vi "Proyecto_KevinLopez.vi"() -> ()   [LabVIEW 2020]
uses:
  <vilib>/userDefined/High Color/IMAQdx.ctl
  <vilib>/vision/driver/NI_Vision_Acquisition_Software.lvlib
  <vilib>/vision/NI_Vision_Development_Module.lvlib
panel:
  out "Amarillo":bool
  out "Rojo":bool
  out "Azul":bool
  out "Verde":bool
  out "Color Spectrum":dbl[](array[numeric]) format="%.2f"
  in  "Color Sensitivity":u32(ring) items=["Low", "Medium", "High"]
  in  "Session In":T1
  in  "stop":bool
  out "Image":T2(plugin-control)
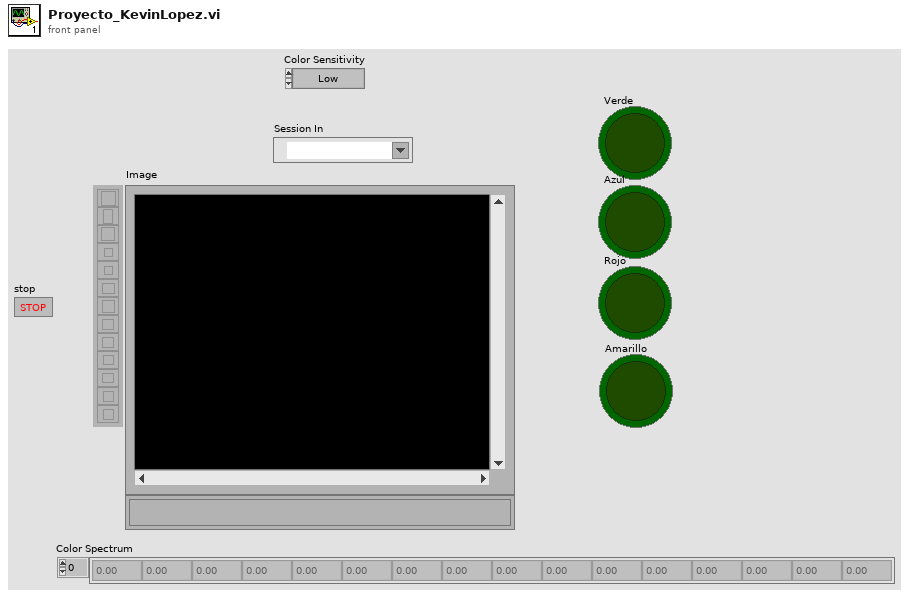
[diagram p1: front panel]
types:
  T1 = typedef "IMAQdx.ctl" = refnum<k21>
  T2 = typedef "IMAQ Image.ctl" = refnum<image>
  T3 = cluster{"Global Rectangle":i32[], "Contours":cluster{"Contour Type":u32, "ROI Type":u32, "Points":i32[]}[]}
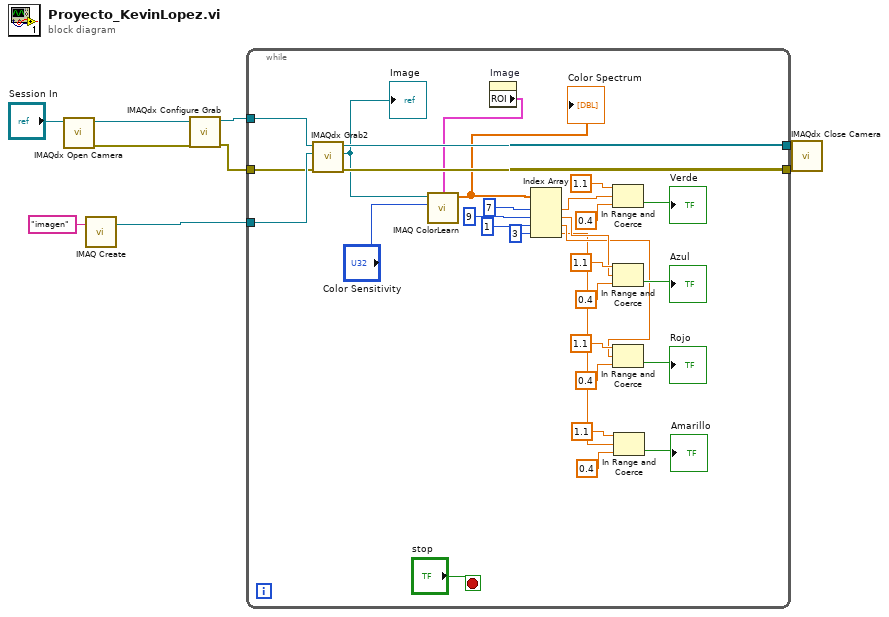
[diagram p0: block diagram]
diagram:
  n1 = call <vilib>:"IMAQdx Open Camera.vi"("Session In"="Session In") -> ("error out"=w8:errorcluster, "Session Out"=w9:T1)  [unwired: 9 in]
  n2 = call "IMAQ Create"("Image Name"="imagen") -> ("New Image"=w6:T2)  [unwired: 4 in, 1 out]
  n3 = call <vilib>:"IMAQdx Configure Grab.vi"("error in"=w8, "Session In"=w9) -> ("error out"=w5:errorcluster, "Session Out"=w4:T1)  [unwired: 8 in]
  n4 = while {
    tunnel: w6 -> [w39]
    tunnel: w5 -> [w38]
    tunnel: w4 -> [w37]
    tunnel: [w34] -> w3
    tunnel: [w36] -> w2
    stop <- "stop" stop-if-true
    n5 = call <vilib>:"IMAQdx Grab2.vi"("error in"=w38, "Image In"=w39, "Session In"=w37) -> ("error out"=w36:errorcluster, "Image Out"=w33:T2, "Session Out"=w34:T1)  [unwired: 5 in, 1 out]
    "Image" <- w33
    n6 = property on="Image" class="ImageControl"() -> ("ROI"=w31:T3)  [unwired: 2 in, 2 out]
    n7 = call "IMAQ ColorLearn"("ROI Descriptor"=w31, "Image"=w33, "Color Sensitivity"="Color Sensitivity") -> ("Color Spectrum"=w27:dbl[])  [unwired: 5 in, 1 out]
    "Color Spectrum" <- w27
    n8 = Index Array(array=w27, index #1=7 ("index"), index #2=9 ("index"), index #3=1 ("index"), index #4=3 ("index")) -> (element #1=w25:dbl, element #2=w14:dbl, element #3=w12:dbl, element #4=w11:dbl)
    n9 = In Range and Coerce(upper limit=1.1, x=w25, lower limit=0.4) -> (In Range?=→"Verde":bool)  [unwired: 1 out]
    n10 = In Range and Coerce(upper limit=1.1, x=w14, lower limit=0.4) -> (In Range?=→"Azul":bool)  [unwired: 1 out]
    n11 = In Range and Coerce(upper limit=1.1, x=w12, lower limit=0.4) -> (In Range?=→"Rojo":bool)  [unwired: 1 out]
    n12 = In Range and Coerce(upper limit=1.1, x=w11, lower limit=0.4) -> (In Range?=→"Amarillo":bool)  [unwired: 1 out]
  }
  n13 = call <vilib>:"IMAQdx Close Camera.vi"("error in"=w2, "Session In"=w3) -> ()  [unwired: 9 in, 1 out]
